vi "GenerateAttackablePosition_King.vi"(1 "Black/White Turn (T/F)":bool, 2 "Board":i32[][](array[numeric])=[[-3, -5, -4, -1, -2, -4, -5, -3], [-6, -6, -6, -6, -6, -6, -6, -6], [0, 0, 0, 0, 0, 0, 0, 0], [0, 0, 0, 0, 0, 0, 0, 0], [0, 0, 0, 0, 0, 0, 0, 0], [0, 0, 0, 0, 0, 0, 0, 0], [6, 6, 6, 6, 6, 6, 6, 6], [3, 5, 4, 1, 2, 4, 5, 3]], 3 "pieceIndex":i32) -> (0 "AttackablePosition":bool[][](array[boolean]))   [LabVIEW 2014]
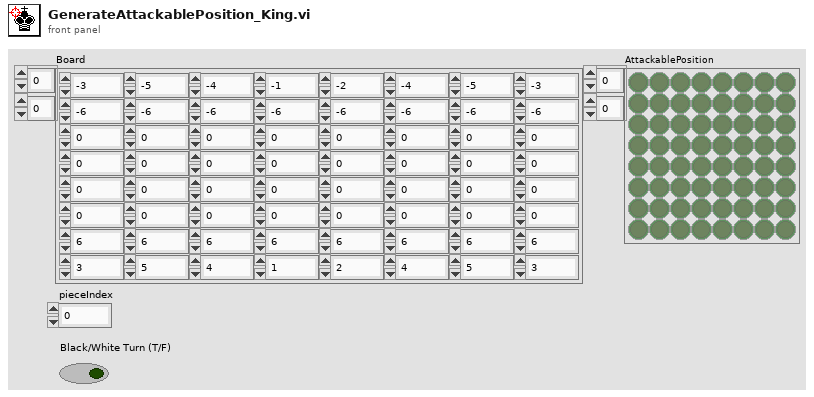
[diagram p1: front panel]
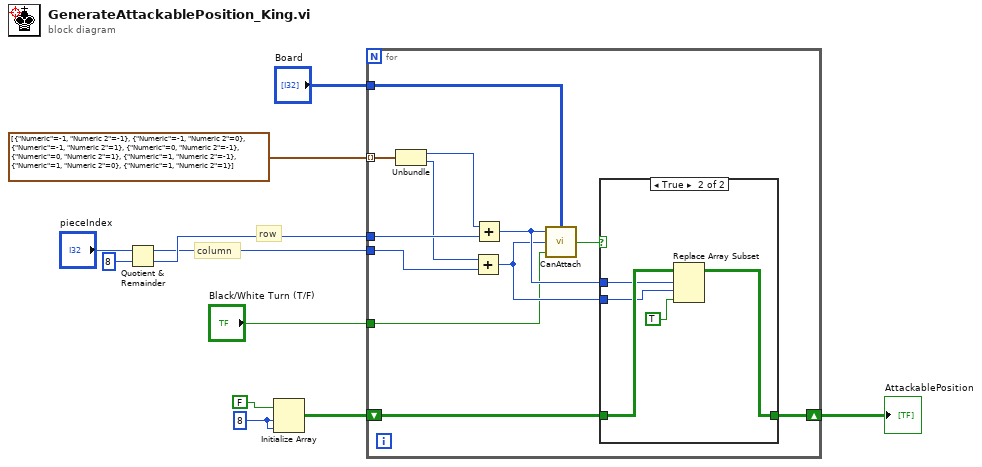
[diagram p0: block diagram]
diagram:
  w4 = 8 ("dimension size")
  # "column"
  # "row"
  n1 = Quotient & Remainder(x="pieceIndex", y=8) -> (x-y*floor(x/y)=w7:i32, floor(x/y)=w8:i32)
  n2 = Initialize Array(FALSE, w4, w4) -> (w2:bool[][])
  n3 = for {
    tunnel: cluster{"Numeric":i32, "Numeric 2":i32}[] [{"Numeric"=-1, "Numeric 2"=-1}, {"Numeric"=-1, "Numeric 2"=0}, {"Numeric"=-1, "Numeric 2"=1}, {"Numeric"=0, "Numeric 2"=-1}, {"Numeric"=0, "Numeric 2"=1}, {"Numeric"=1, "Numeric 2"=-1}, {"Numeric"=1, "Numeric 2"=0}, {"Numeric"=1, "Numeric 2"=1}] ("Array") -> [w23] mode=indexing
    tunnel: w8 -> [w22]
    tunnel: w7 -> [w20]
    shift-right: [w12] -> w5
    shift-left: w2 -> [w13]
    tunnel: "Board" -> [w17]
    tunnel: "Black/White Turn (T/F)" -> [w14]
    n4 = Unbundle(w23) -> ("Numeric"=w21:i32, "Numeric 2"=w19:i32)
    n5 = Add(x=w19, y=w20) -> (x+y=w15:i32)
    n6 = Add(x=w21, y=w22) -> (x+y=w16:i32)
    n7 = call "CanAttach.vi"("Board"=w17, "Black/White Turn (T/F)"=w14, "Column"=w15, "Row"=w16) -> ("Boolean"=w18:bool)
    n8 = case shown="True" w18 {
      tunnel: w16 -> [_ w28]
      tunnel: w15 -> [_ w27]
      tunnel: w13 -> [w24 w29]
      tunnel: [w24 w26] -> w12
      frame False {
      }
      frame True {
        n9 = Replace Array Subset(array=w29, new element=TRUE ("new element/subarray"), index (row)=w28, index (col)=w27) -> (w26:bool[][])
      }
    }
  }
  "AttackablePosition" <- w5
